vi "Write Variant DB.vi"(8 "error in (no error)":errorcluster, 10 "Variant DB":variant, 11 "SeqGen Step Dictionary in":refnum<class "SeqGen Step Dictionary.lvclass">) -> (0 "error out":errorcluster, 3 "SeqGen Step Dictionary out":refnum<class "SeqGen Step Dictionary.lvclass">)   [LabVIEW 2018, in "SeqGen Step Database.lvlib" / "SeqGen Step Dictionary.lvclass"]
uses:
  SeqGen Step Dictionary.lvclass
  SeqGen Step Dictionary.lvclass/SeqGen Step Dictionary.ctl
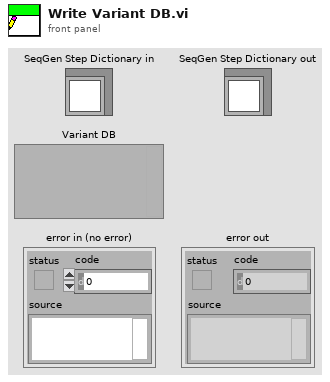
[diagram p1: front panel]
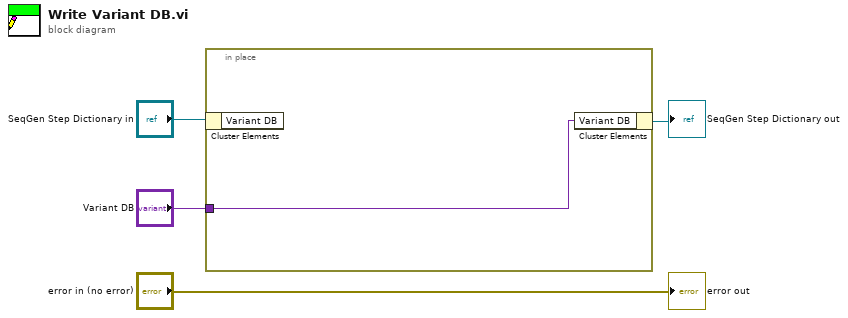
[diagram p0: block diagram]
diagram:
  n1 = in-place {
    in-place-border: "Variant DB" -> [w5]
    n2 = in-place-cluster #1("SeqGen Step Dictionary in") -> ()  [unwired: 1 out]
    n3 = in-place-cluster #1("Variant DB"=w5) -> (→"SeqGen Step Dictionary out":refnum<class "SeqGen Step Dictionary.lvclass">)
  }
  "error out" <- "error in (no error)"
